vi "Tx Streaming (Host)(Single channel).vi"() -> ()   [LabVIEW 2019]
doc: "This template is for the Simple NI-USRP Streaming design, a design that shows the basics of streaming data to and from an NI USRP-294x/295x device. Refer to the block diagram for more information about how to use this template."
uses:
  <instrlib>/niUSRP/niUSRP Write Tx Data (CDB).vi
  <vilib>/Utility/file.llb/Read From Spreadsheet File (DBL).vi
panel:
  in  "Carrier Frequency":dbl=2400000000.0 format="%#.8p"
  in  "IQ Rate":dbl=500000.0 format="%#.8p"
  out "Data":dbl[](graph)
  in  "Upload Chunk Size":i32=100000
  in  "stop":bool
  in  "Set Gain":bool
  in  "Gain":dbl=20.0
  in  "device name":refnum<k15>="192.168.10.2"
  in  "file (use dialog)":path=path "C:/Users/Burton/Desktop/软件定义平台/G-64.txt"
  # "Configure Tx Signal"
  # "Front Panel Steps:\n\n1)  Select the file path of the text file you would like to use for the signal generation in the \"file (use dialog)\" control.\n2)   Enter the name of your device in the \"device name\" control.\n3)  While the code is running, adjust the gain by setting the value in the \"Gain\" control and pushing the \"Set Gain\" button.\nNote:  Make sure to keep the Upload Chunk Size, samples value around 100,000 for 8MS/s IQ Rate."
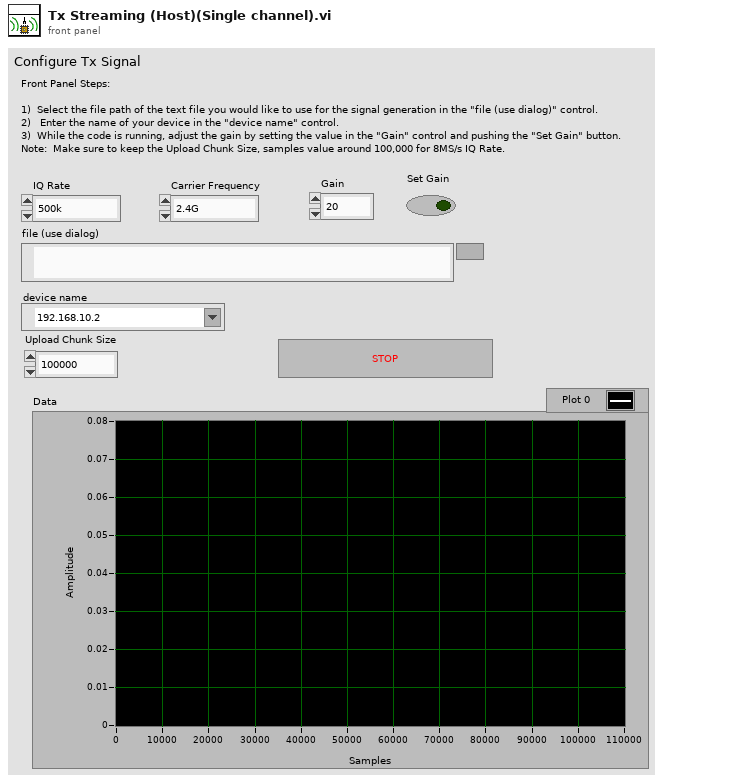
[diagram p1: front panel]
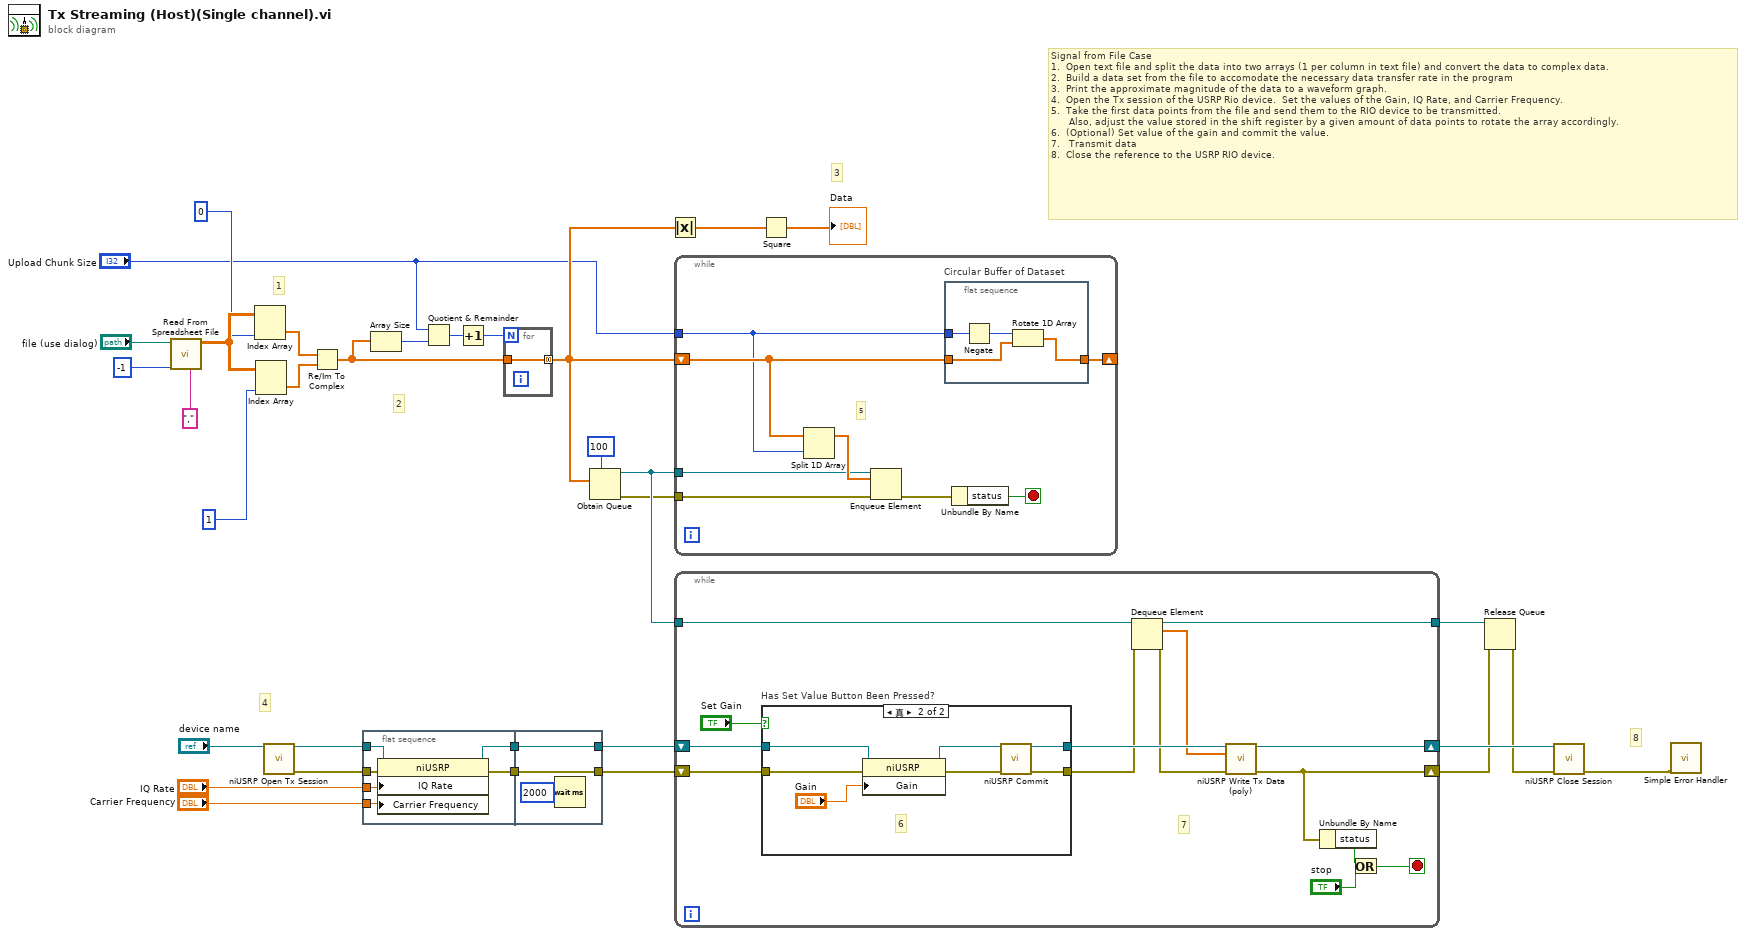
[diagram p0: block diagram]
diagram:
  # "4"
  # "1"
  # "3"
  # "2"
  # "Signal from File Case\n1.  Open text file and split the data into two arrays (1 per column in text file) and convert the data to complex data.\n2.  Build a data set from the file to accomodate the necessary data transfer rate in the program\n3.  Print the approximate magnitude of the data to a waveform graph.\n4.  Open the Tx session of the USRP Rio device.  Set the values of the Gain, IQ Rate, and Carrier Frequency.\n5.  Take the first data points from the file and send them to the RIO device to be transmitted.  \n      Also, adjust the value stored in the shift register by a given amount of data points to rotate the array accordingly.\n6.  (Optional) Set value of the gain and commit the value.\n7.   Transmit data\n8.  Close the reference to the USRP RIO device."
  # "8"
  n1 = call-poly <vilib>:"Read From Spreadsheet File.vi"("delimiter (\\t)"="," ("delimiter (\\t)"), "number of rows (all:-1)"=-1, "file path (dialog if empty)"="file (use dialog)") -> ("all rows"=w16:dbl[][])  [unwired: 4 in, 4 out]
  n2 = Index Array(array=w16, index (col)=0 ("disabled index (col)")) -> (element=w14:dbl[])  [unwired: 1 in]
  n3 = Index Array(array=w16, index (col)=1 ("disabled index (col)")) -> (element=w15:dbl[])  [unwired: 1 in]
  n4 = call <instrlib>:"niUSRP Open Tx Session.vi"("device names"="device name") -> ("session handle out"=w1:refnum<k15>, "error out"=w28:errorcluster)  [unwired: 13 in]
  n5 = Re/Im To Complex(1:w15, 2:w14) -> (0:w10:cdb[])
  n6 = flat-sequence {
    tunnel: w28 -> [w39]
    tunnel: w1 -> [w37]
    tunnel: "IQ Rate" -> [w35]
    tunnel: "Carrier Frequency" -> [w34]
    tunnel: [w38] -> w5
    tunnel: [w36] -> w4
    tunnel: [w41] -> w26
    tunnel: [w42] -> w27
    tunnel: w5 -> [w42]
    tunnel: w4 -> [w41]
    frame #0 {
      n7 = property class="niUSRP"(reference=w37, error in=w39, "IQ Rate"=w35, "Carrier Frequency"=w34) -> (reference out=w36:refnum<k15>, error out=w38:errorcluster)
    }
    frame #1 {
      n8 = Wait (ms)(milliseconds to wait=u32 2000) -> ()  [unwired: 1 out]
    }
  }
  n9 = Array Size(array=w10) -> (size(s)=w9:i32)
  n10 = Quotient & Remainder(x="Upload Chunk Size", y=w9) -> (floor(x/y)=w7:i32)  [unwired: 1 out]
  n11 = Increment(x=w7) -> (x+1=w6:i32)
  n12 = for {
    N: w6 -> [_]
    tunnel: [w43] -> w11 mode=concatenating
    tunnel: w10 -> [w43]
  }
  n13 = Obtain Queue(max queue size (-1, unlimited)=100, element data type=w11) -> (queue out=w24:refnum<queue>, error out=w23:errorcluster)  [unwired: 3 in, 1 out]
  n14 = Absolute Value(x=w11) -> (abs(x)=w25:dbl[])
  n15 = while {
    tunnel: w24 -> [w45]
    tunnel: w23 -> [w44]
    shift-right: [w49] -> _
    shift-left: w11 -> [w48]
    tunnel: "Upload Chunk Size" -> [w46]
    stop <- w51 stop-if-true
    # "5"
    n16 = Split 1D Array(array=w48, index=w46) -> (first subarray=w47:cdb[])  [unwired: 1 out]
    n17 = Enqueue Element(queue=w45, element=w47, error in (no error)=w44) -> (error out=w50:errorcluster)  [unwired: 1 in, 2 out]
    n18 = flat-sequence "Circular Buffer of Dataset" {
      tunnel: [w55] -> w49
      tunnel: w48 -> [w54]
      tunnel: w46 -> [w52]
      frame #0 {
        n19 = Negate(x=w52) -> (-x=w53:i32)
        n20 = Rotate 1D Array(1:w54, 2:w53) -> (0:w55:cdb[])
      }
    }
    n21 = Unbundle By Name(w50) -> ("status"=w51:bool)
  }
  n22 = while {
    shift-right: [w68] -> w18
    shift-left: w27 -> [w67]
    shift-right: [w69] -> w32
    shift-left: w26 -> [w66]
    tunnel: w24 -> [w63]
    tunnel: [w59] -> w22
    stop <- w62 stop-if-true
    # "7"
    n23 = case "Has Set Value Button Been Pressed?" shown="真" "Set Gain" {
      tunnel: [w71 w78] -> w61
      tunnel: [w70 w77] -> w58
      tunnel: w66 -> [w71 w73]
      tunnel: w67 -> [w70 w76]
      frame False {
      }
      frame True {
        # "6"
        n24 = property class="niUSRP"(reference=w73, error in=w76, "Gain"="Gain") -> (reference out=w72:refnum<k15>, error out=w74:errorcluster)
        n25 = call <instrlib>:"niUSRP Commit.vi"("session handle"=w72, "error in (no error)"=w74) -> ("session handle out"=w78:refnum<k15>, "error out"=w77:errorcluster)  [unwired: 12 in]
      }
    }
    n26 = Dequeue Element(queue=w63, error in (no error)=w58) -> (queue out=w59:refnum<queue>, element=w56:cdb[], error out=w57:errorcluster)  [unwired: 1 in, 1 out]
    n27 = call-poly <instrlib>:"niUSRP Write Tx Data (poly).vi"("session handle"=w61, "data"=w56, "error in (no error)"=w57) -> ("session handle out"=w69:refnum<k15>, "error out"=w68:errorcluster)  [unwired: 11 in]
    n28 = Unbundle By Name(w68) -> ("status"=w65:bool)
    n29 = Or(x=w65, y="stop") -> (x .or. y?=w62:bool)
  }
  n30 = Square(x=w25) -> (x^2=→"Data":dbl[])
  n31 = Release Queue(queue=w22, error in (no error)=w18) -> (error out=w17:errorcluster)  [unwired: 1 in, 2 out]
  n32 = call <instrlib>:"niUSRP Close Session.vi"("session handle"=w32, "error in (no error)"=w17) -> ("error out"=w19:errorcluster)  [unwired: 13 in]
  n33 = call <vilib>:"Simple Error Handler.vi"("error in (no error)"=w19) -> ()  [unwired: 4 in, 5 out]
